vi "Get Match ID Example.vi"() -> ()   [LabVIEW 2025]
panel:
  in  "OK Button":bool
  out "return value 4":string
  in  "stop":bool
  out "return value 3":string
  out "return value 2":string
  out "s? t:f":errorcluster
  out "return value":string
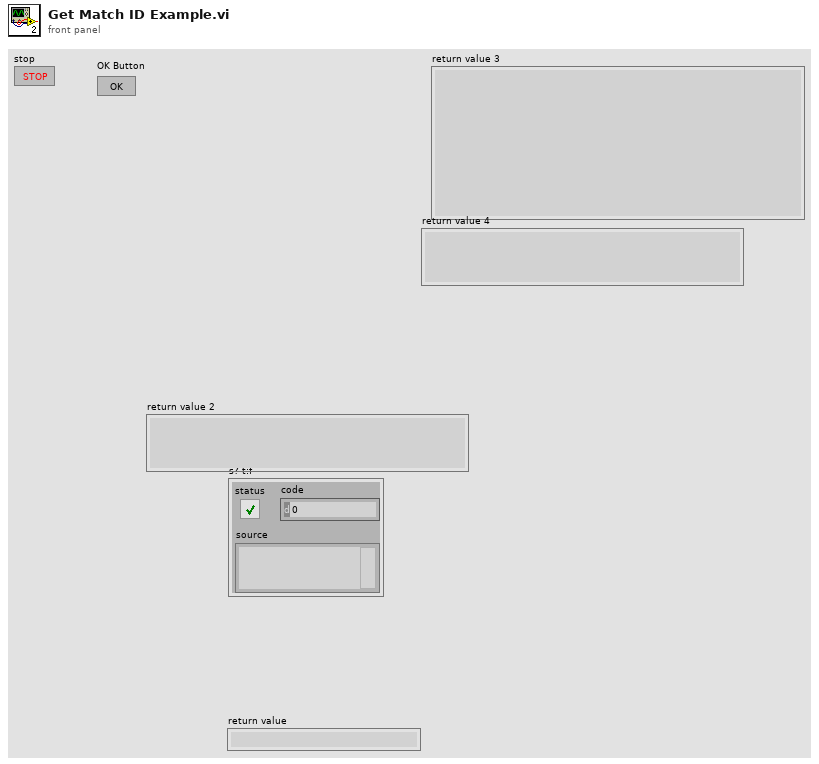
[diagram p1: front panel]
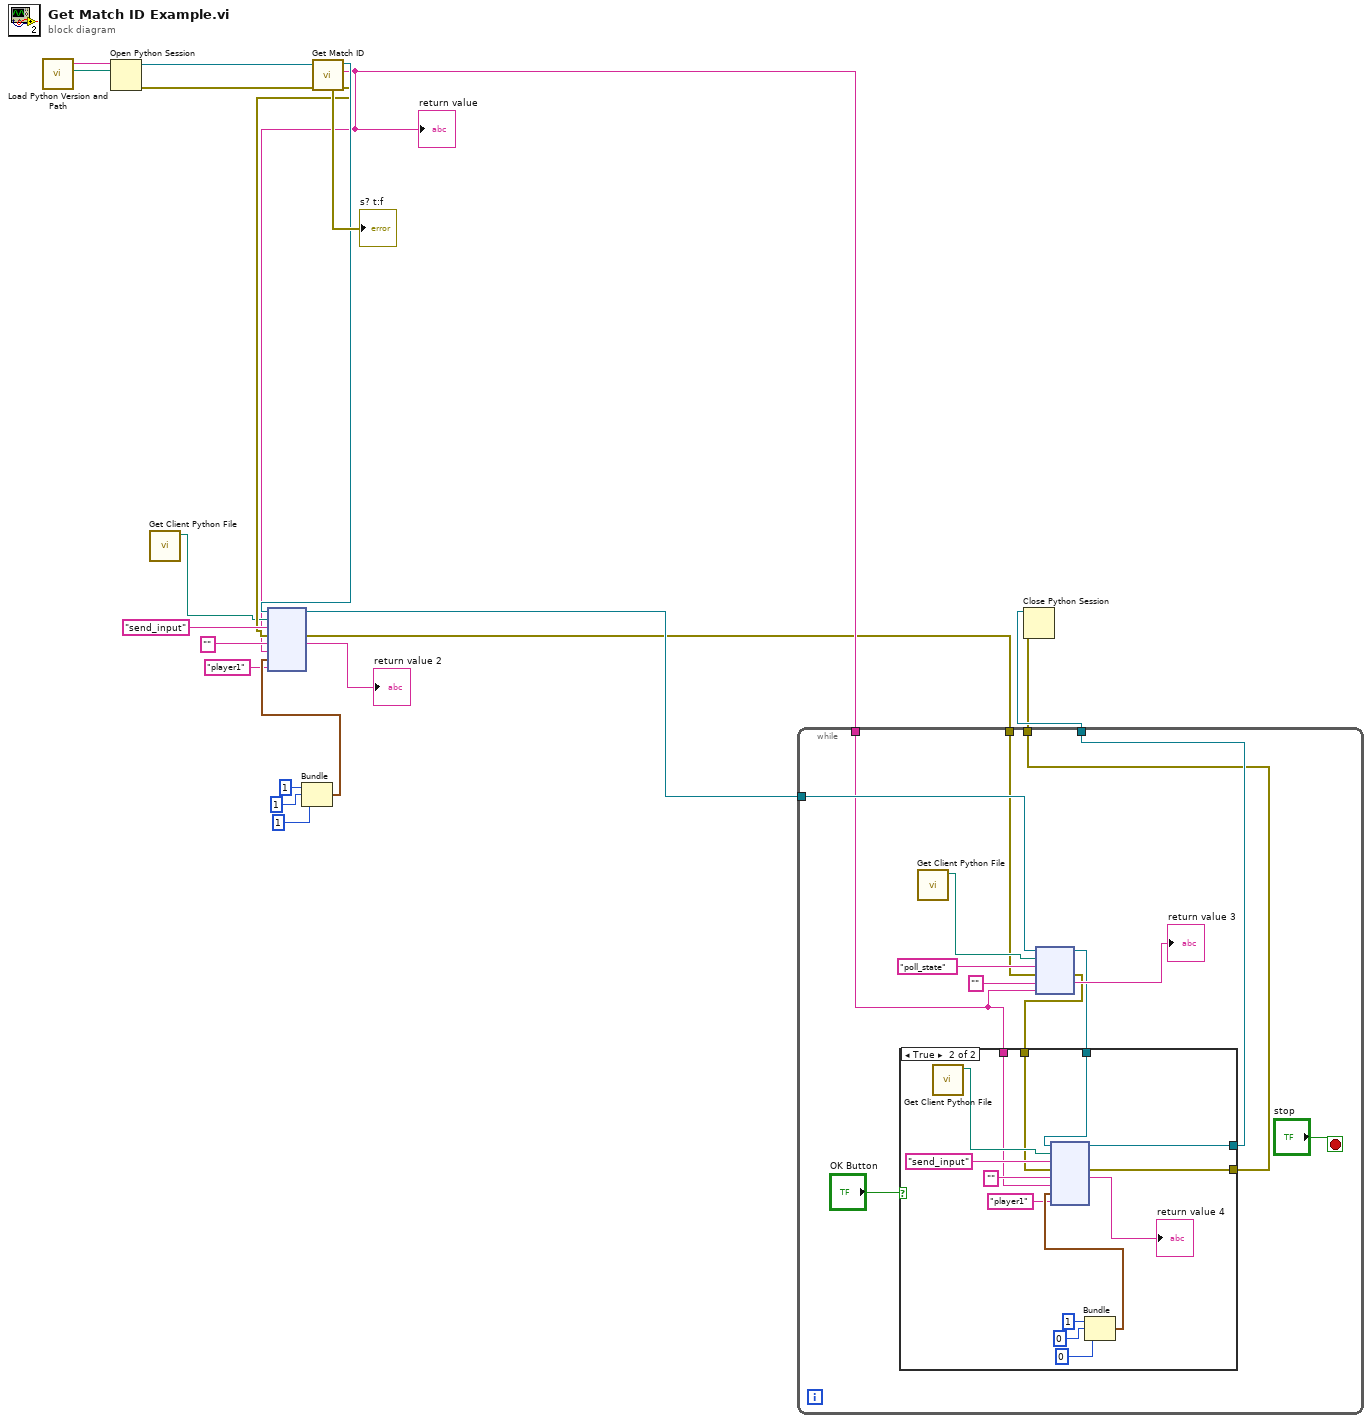
[diagram p0: block diagram]
diagram:
  n1 = call "Load Python Version and Path.vi"() -> ("path"=w20:path, "version"=w21:string)  [unwired: 10 in]
  n2 = Open Python Session(python version=w21, python path=w20) -> (session out=w19:refnum<k35>, error out=w18:errorcluster)  [unwired: 1 in]
  n3 = call "Get Client Python File.vi"() -> ("appended path"=w6:path)  [unwired: 11 in]
  n4 = Bundle(1, 1, 1) -> (w11:cluster{i32, i32, i32})  [unwired: 1 in]
  n5 = call "Get Match ID.vi"("Refnum in"=w19, "error in (no error)"=w18) -> ("Refnum out"=w13:refnum<k35>, "return value"=w5:string, "is_ok"=→"s? t:f":errorcluster, "error out"=w12:errorcluster)  [unwired: 5 in]
  "return value" <- w5
  n6 = node(w13, w6, "send_input" ("function name"), w12, "", w5, w11, "player1") -> (w4:refnum<k35>, w3:errorcluster, →"return value 2":string)  [unwired: 3 in, 2 out]
  n7 = while {
    tunnel: w5 -> [w22]
    tunnel: w4 -> [w31]
    tunnel: w3 -> [w30]
    tunnel: [w25] -> w2
    tunnel: [w24] -> w1
    stop <- "stop" stop-if-true
    n8 = call "Get Client Python File.vi"() -> ("appended path"=w34:path)  [unwired: 11 in]
    n9 = node(w31, w34, "poll_state" ("function name"), w30, "", w22) -> (w26:refnum<k35>, w27:errorcluster, →"return value 3":string)  [unwired: 1 in, 2 out]
    n10 = case shown="True" "OK Button" {
      tunnel: w27 -> [w36 w42]
      tunnel: w26 -> [w35 w41]
      tunnel: [w35 w40] -> w25
      tunnel: [w36 w39] -> w24
      tunnel: w22 -> [_ w38]
      frame False {
      }
      frame True {
        n11 = call "Get Client Python File.vi"() -> ("appended path"=w43:path)  [unwired: 11 in]
        n12 = Bundle(1, 0, 0) -> (w47:cluster{i32, i32, i32})  [unwired: 1 in]
        n13 = node(w41, w43, "send_input" ("function name"), w42, "", w38, w47, "player1") -> (w40:refnum<k35>, w39:errorcluster, →"return value 4":string)  [unwired: 3 in, 2 out]
      }
    }
  }
  n14 = Close Python Session(session in=w2, error in=w1) -> ()  [unwired: 1 out]
